vi "TinySpeakServer.vi"() -> ()   [LabVIEW 2010]
panel:
  out "text sent ascii":string
  out "text sent":string
  out "name":string
  in  "stop":bool
  out "text received":string
  in  "port":u16=9999
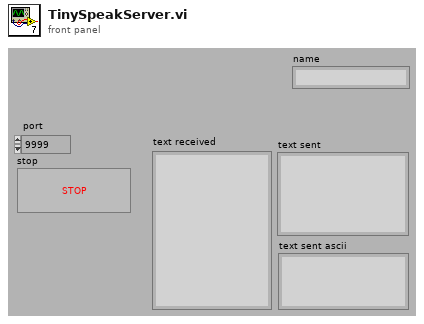
[diagram p1: front panel]
types:
  T1 = enum16{"Standard", "Buffered", "CRLF", "Immediate"}
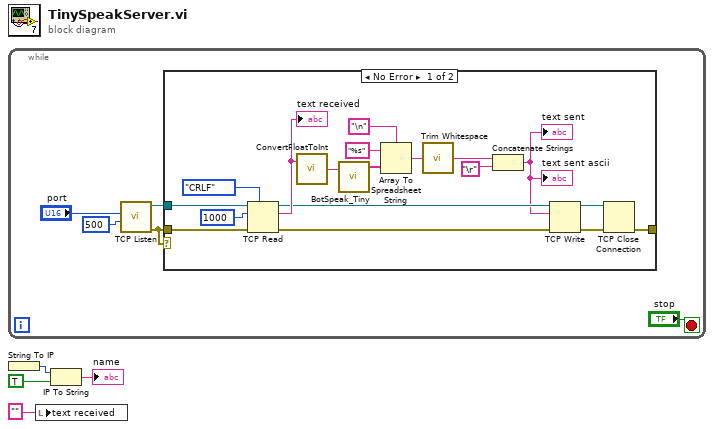
[diagram p0: block diagram]
diagram:
  n1 = while {
    stop <- "stop" stop-if-true
    n2 = call <vilib>:"TCP Listen.vi"("timeout ms (wait forever: -1)"=500, "port"="port") -> ("error out"=w7:errorcluster, "connection ID"=w8:refnum<k5>)  [unwired: 6 in, 2 out]
    n3 = case shown="No Error" w7 {
      tunnel: w7 -> [w27 _]
      tunnel: w8 -> [w26 _]
      tunnel: [w14 _] -> _
      frame No Error {
        n4 = TCP Read(connection ID=w26, bytes to read=1000, error in (no error)=w27, 7:T1."CRLF" ("mode (standard)")) -> (connection ID out=w18:refnum<k5>, data out=w23:string, error out=w17:errorcluster)  [unwired: 1 in]
        "text received" <- w23
        n5 = call <userlib>:"ConvertFloatToInt.vi"("To Send in"=w23) -> ("To Send out"=w22:string)  [unwired: 1 in]
        n6 = call <userlib>:"BotSpeak_Tiny.vi"("URAPI"=w22) -> ("Tiny Lines"=w20:string[])  [unwired: 1 in, 2 out]
        n7 = Array To Spreadsheet String(delimiter (Tab)="\n", array=w20, 3:"%s" ("delimiter (Tab)")) -> (spreadsheet string=w21:string)
        n8 = call <vilib>:"Trim Whitespace.vi"("string"=w21) -> ("trimmed string"=w12:string)  [unwired: 1 in]
        n9 = Concatenate Strings(w12, "\r") -> (w10:string)
        "text sent" <- w10
        "text sent ascii" <- w10
        n10 = TCP Write(connection ID=w18, data in=w10, error in (no error)=w17) -> (connection ID out=w15:refnum<k5>, error out=w16:errorcluster)  [unwired: 1 in, 1 out]
        n11 = TCP Close Connection(connection ID=w15, error in (no error)=w16) -> (error out=w14:errorcluster)  [unwired: 1 in, 1 out]
      }
      frame Error {
      }
    }
  }
  n12 = String To IP() -> (0:w3:u32)  [unwired: 1 in]
  n13 = local write "text received"("" ("text received")) -> ()
  n14 = IP To String(1:TRUE ("dot notation? (F)"), 2:w3) -> (0:→"name":string)
